vi "Sequence Configurator.vi"() -> ()   [LabVIEW 2024]
doc: "Use this to configure the order of the tests in <project root>/Tests."
uses:
  <vilib>/addons/_JKI Toolkits/State Machine/_JKI_lib_State_Machine.llb/Select State(s)_err__jki_lib_state_machine.vi
  <vilib>/addons/_JKI Toolkits/State Machine/_JKI_lib_State_Machine.llb/Periodic Trigger__ogtk__JKI-SM__jki_lib_state_machine.vi
  <userlib>/_OpenG.lib/file/file.llb/Convert File Extension (String)__ogtk.vi
  <vilib>/Utility/file.llb/Write Delimited Spreadsheet (string).vi
  <userlib>/_OpenG.lib/file/file.llb/openg_file.lvlib
  <userlib>/_OpenG.lib/appcontrol/appcontrol.llb/openg_application_control.lvlib
panel:
  in  "Sequence Name":string
  in  "Close Button":bool
  in  "Save Button":bool
  in  "Test Case Order":i32(listbox)
  out "error out":errorcluster
  in  "error in":errorcluster
  # "SEQUENCE CONFIGURATOR"
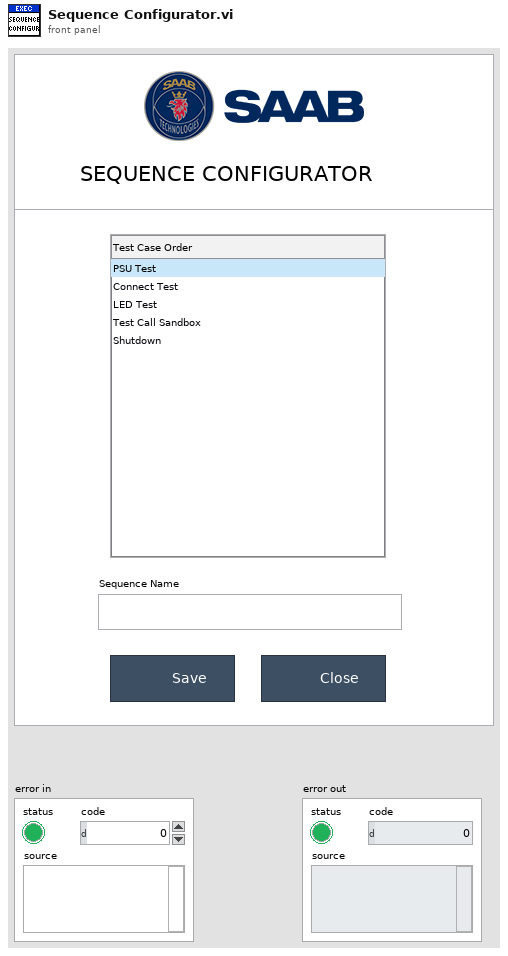
[diagram p1: front panel]
types:
  T1 = enum32{"Invalid", "Standard", "Closed", "Hidden", "Minimized", "Maximized"}
  T2 = enum32{"invalid app kind", "Development System", "Run Time System", "Student Edition", "Embedded LabVIEW", "Evaluation", "Custom"}
  T3 = enum8{"Enabled", "Disabled", "Disabled and Grayed Out"}
  T4 = cluster{"Core":cluster{"Current VI Reference":refnum<vi>, "Close Panel on Exit?":bool}, "Test Case Array":string[], "Sequence Name":string}
  T5 = cluster{"Current VI Reference":refnum<vi>, "Close Panel on Exit?":bool}
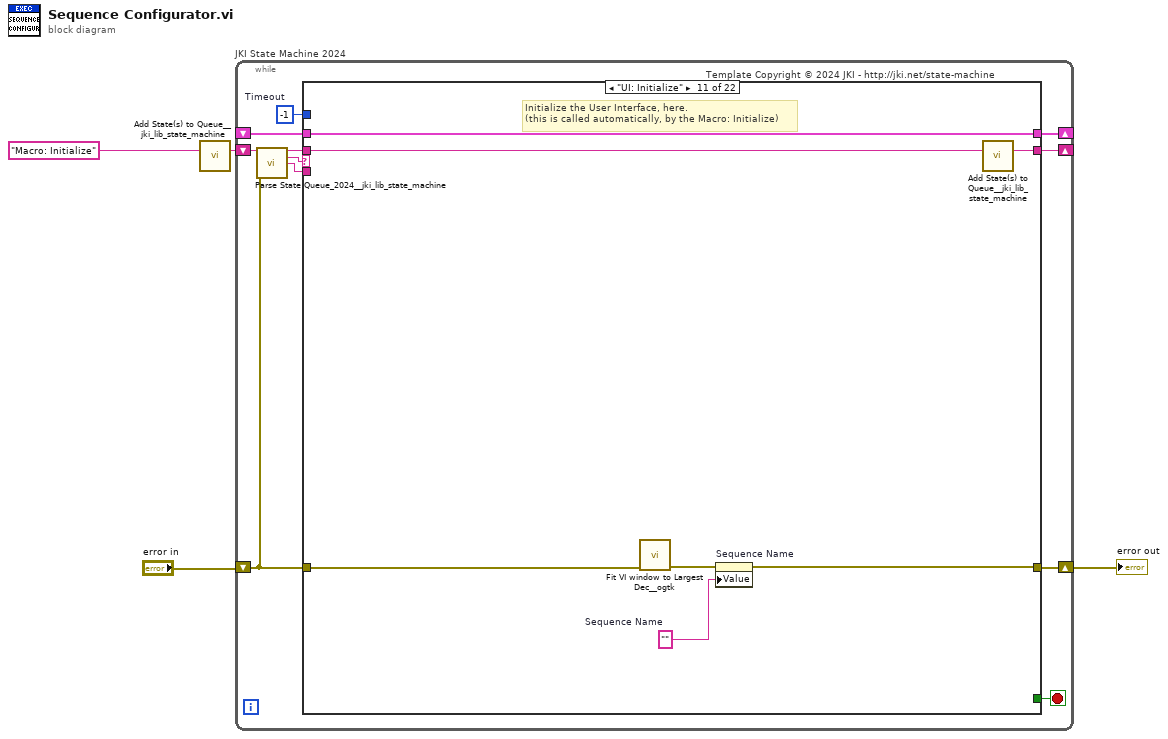
[diagram p0: block diagram]
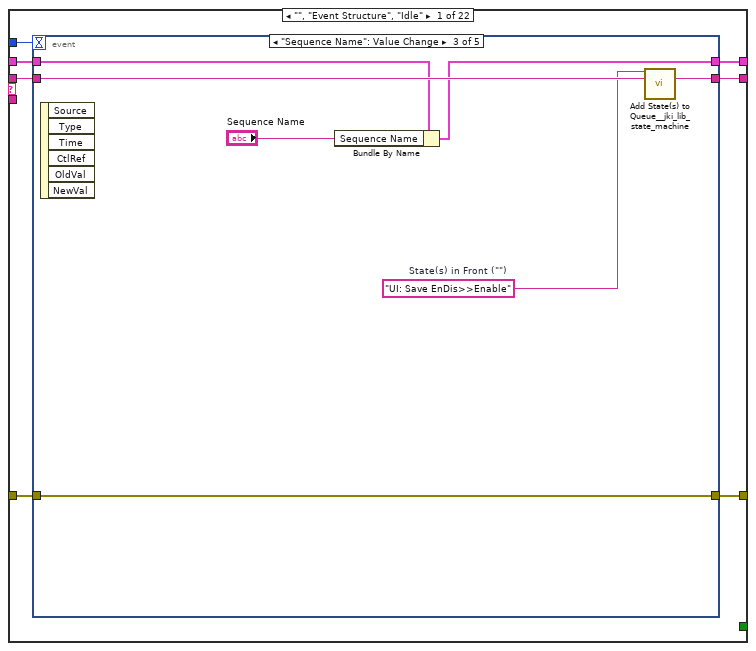
[diagram p2: hidden frame]
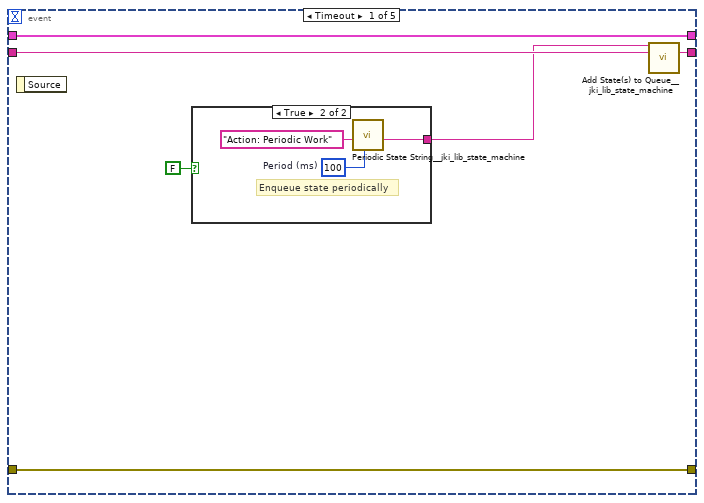
[diagram p3: hidden frame]
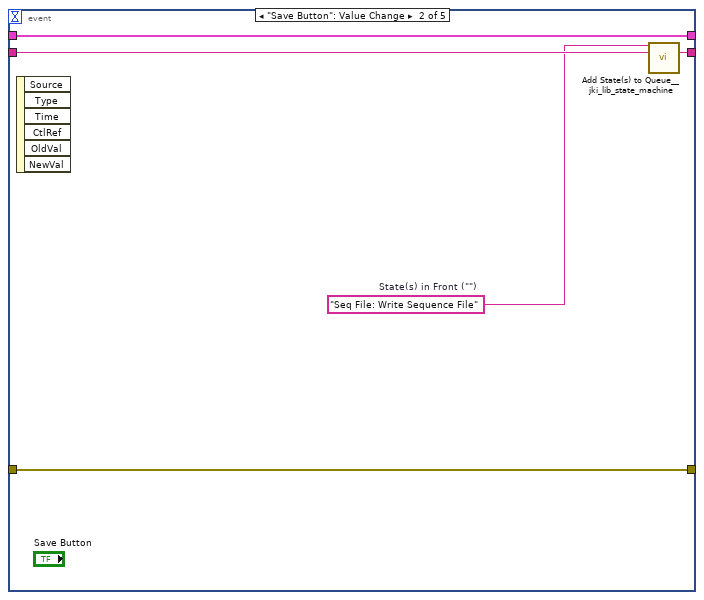
[diagram p5: hidden frame]
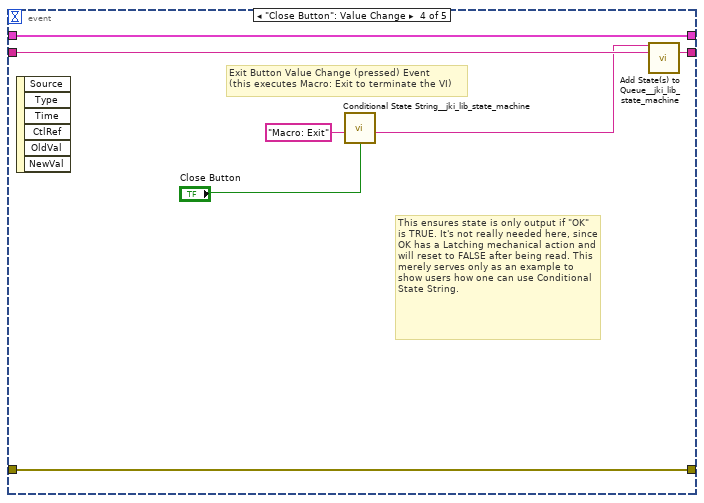
[diagram p6: hidden frame]
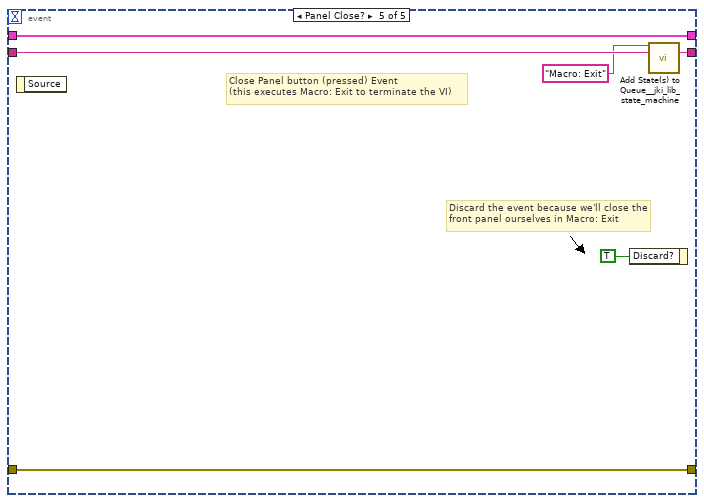
[diagram p7: hidden frame]
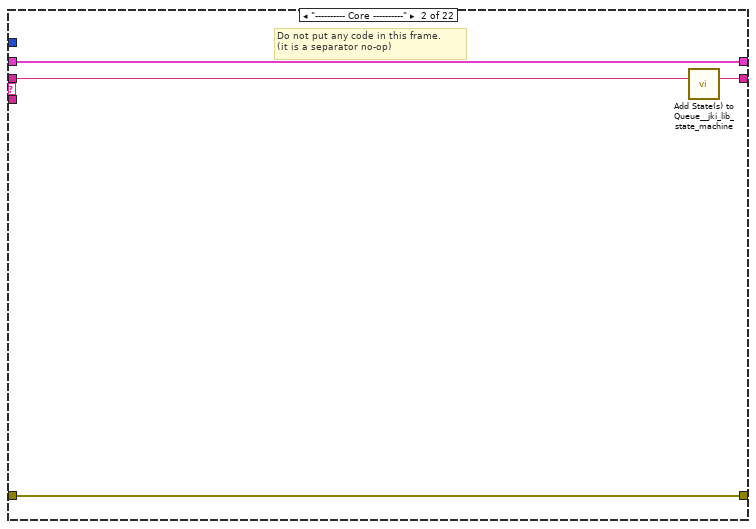
[diagram p8: hidden frame]
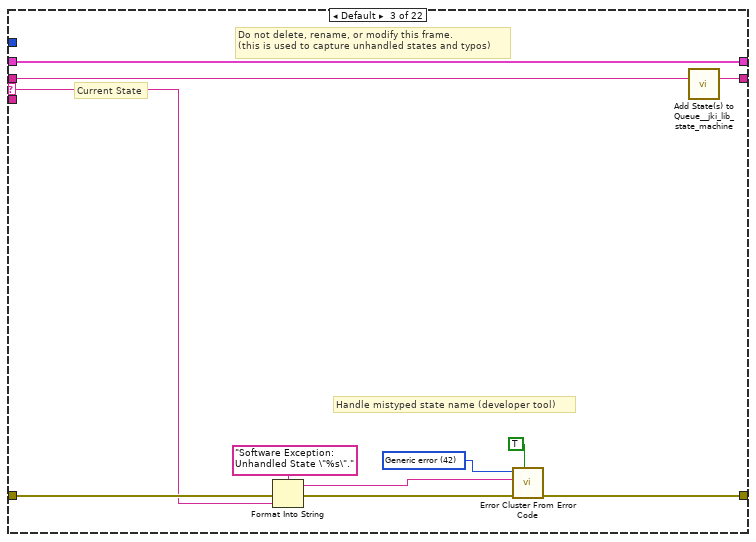
[diagram p9: hidden frame]
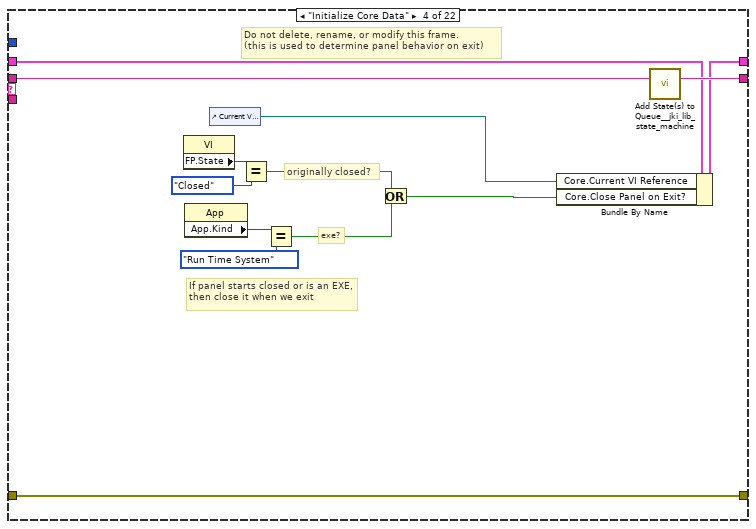
[diagram p10: hidden frame]
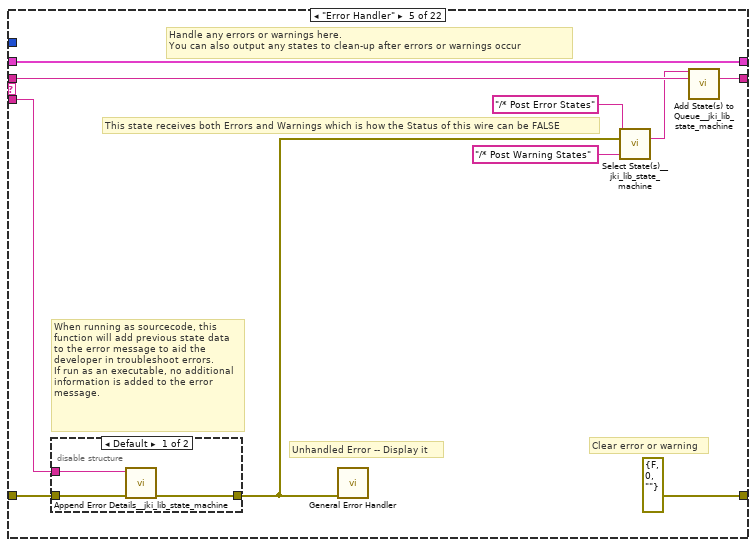
[diagram p11: hidden frame]
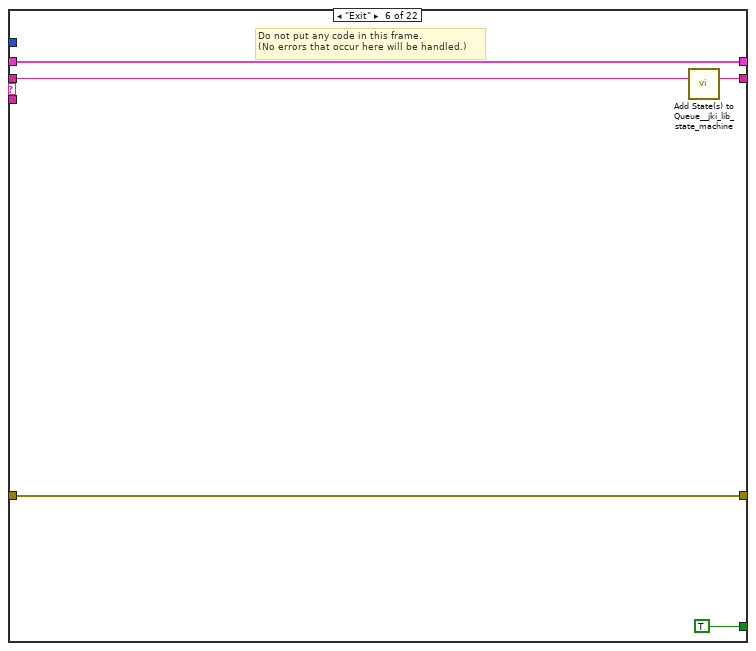
[diagram p13: hidden frame]
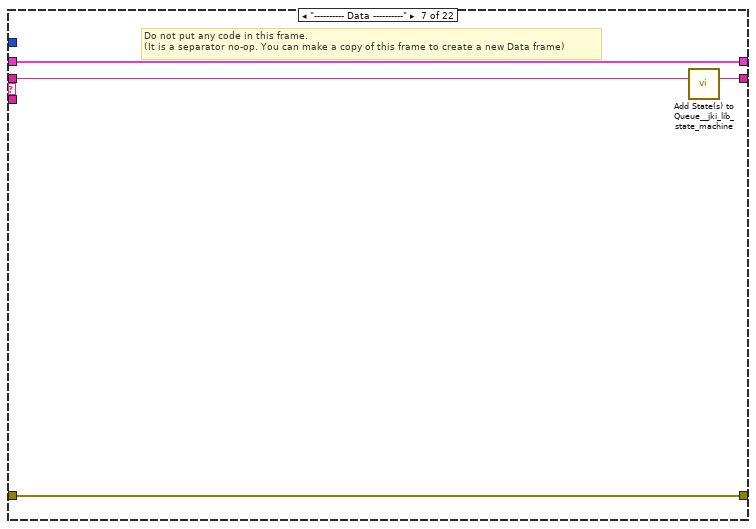
[diagram p14: hidden frame]
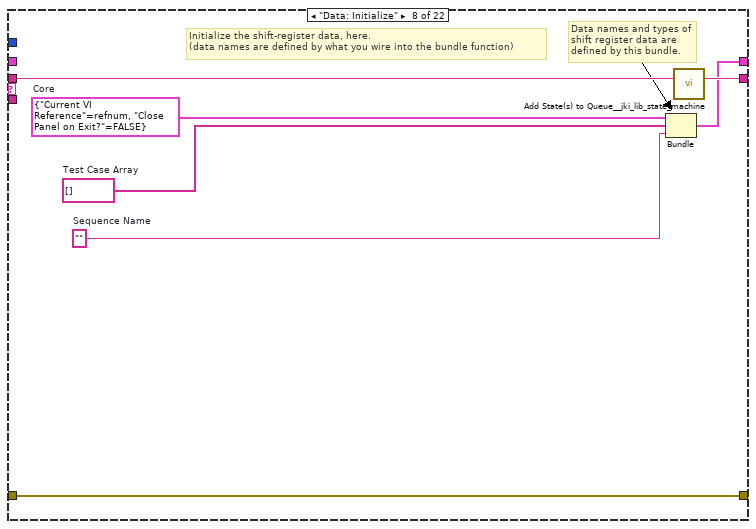
[diagram p15: hidden frame]
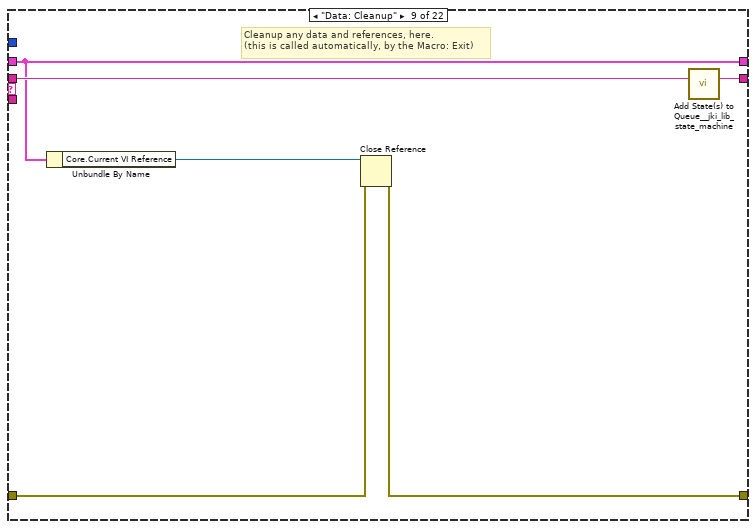
[diagram p16: hidden frame]
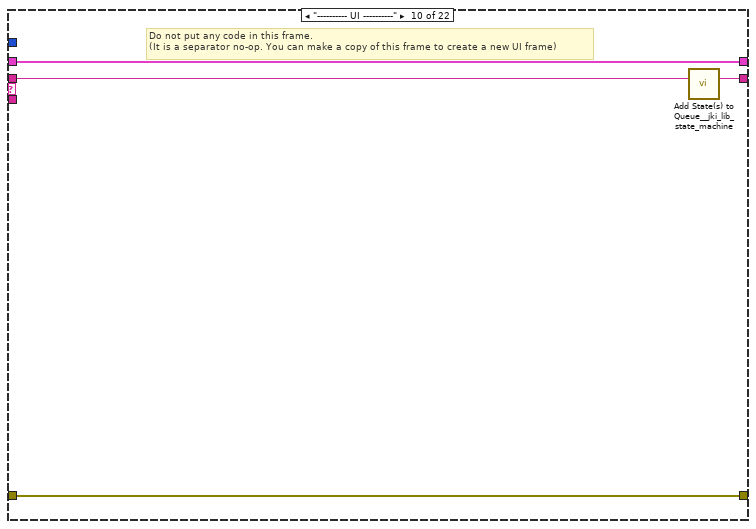
[diagram p17: hidden frame]
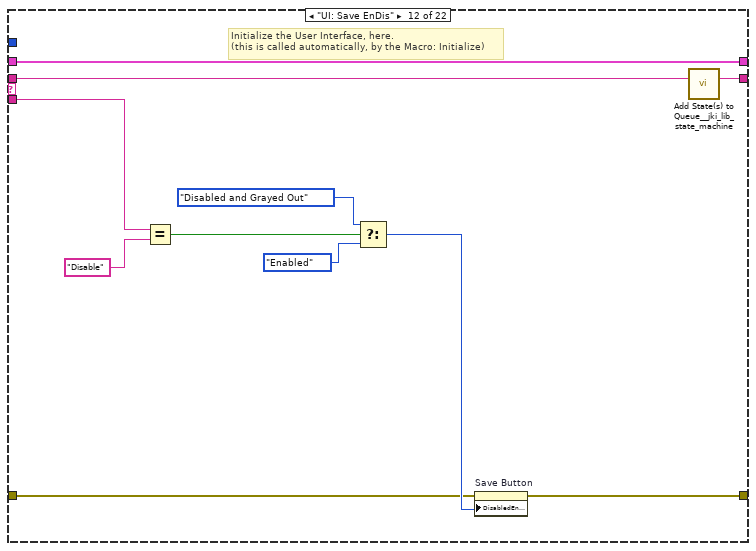
[diagram p18: hidden frame]
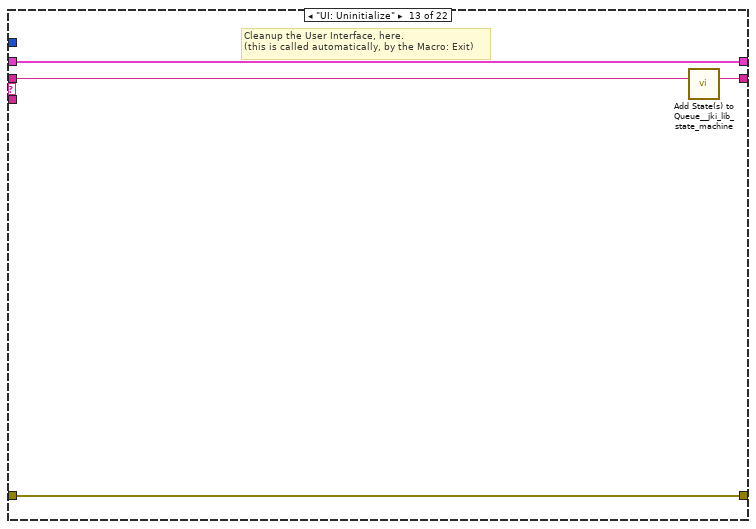
[diagram p19: hidden frame]
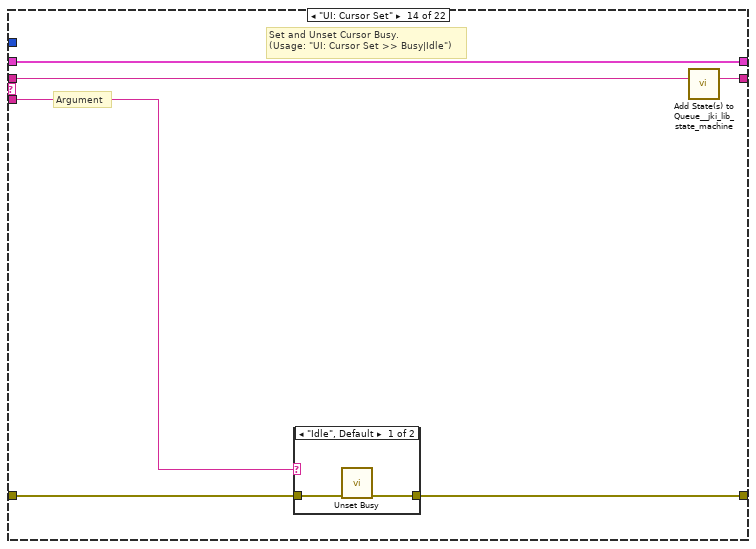
[diagram p20: hidden frame]
diagram:
  n1 = call <vilib>:"Add State(s) to Queue__jki_lib_state_machine.vi"("State(s) in (\"\")"="Macro: Initialize") -> ("States Out"=w4:string)  [unwired: 14 in]
  n2 = while "JKI State Machine 2024" {
    shift-right: [w8] -> _
    shift-left: _ -> [w7]
    shift-right: [w11] -> w1
    shift-left: "error in" -> [w5]
    shift-right: [w10] -> _
    shift-left: w4 -> [w12]
    stop <- w9 stop-if-true
    w6 = -1  # Timeout
    # "Template Copyright © 2024 JKI - http://jki.net/state-machine"
    n3 = call <vilib>:"Parse State Queue_2024__jki_lib_state_machine.vi"("State Queue"=w12, "Error In (no error)"=w5) -> ("Remaining States"=w14:string, "Current State"=w15:string, "Arguments"=w13:string)  [unwired: 11 in]
    n4 = case shown="\"UI: Initialize\"" w15 {
      selector: w15 -> [_ _ w61 _ _ _ _ _ _ _ _ _ _ _ _ _ _ _ _ _ _ _]
      tunnel: w14 -> [w22 w60 w65 w84 w94 w103 w107 w114 w120 w124 w131 w142 w146 w152 w163 w232 w237 w246 w250 w262 w273 w286]
      tunnel: w13 -> [_ _ _ _ w89 _ _ _ _ _ _ w132 _ w147 w157 _ _ _ _ _ _ _]
      tunnel: w7 -> [w20 w57 w63 w77 w91 w101 w104 _ w115 w121 w129 w140 w144 w150 w159 w229 w234 w244 w247 w257 w271 w277]
      tunnel: [w19 w58 w67 w81 errorcluster {"status"=FALSE, "code"=0, "source"=""} ("error out") w100 w105 w111 w116 w122 w127 w133 w143 w148 w160 w230 w235 w241 w248 w260 w266 w282] -> w11
      tunnel: w5 -> [w16 w58 w66 w81 w90 w100 w105 w111 w117 w122 w128 w134 w143 w149 w161 w230 w235 w241 w248 w260 w267 w284]
      tunnel: [w21 w59 w64 w83 w93 w102 w106 w113 w119 w123 w130 w141 w145 w151 w162 w231 w236 w245 w249 w261 w272 w285] -> w10
      tunnel: [_ _ _ _ _ TRUE _ _ _ _ _ _ _ _ _ _ _ _ _ _ _ _] -> w9
      tunnel: [w18 w57 w63 w82 w91 w101 w104 w112 w115 w121 w129 w140 w144 w150 w159 w229 w234 w244 w247 w256 w271 w277] -> w8
      tunnel: w6 -> [w17 _ _ _ _ _ _ _ _ _ _ _ _ _ _ _ _ _ _ _ _ _]
      frame "", "Event Structure", "Idle" {
        n5 = event shown="[2] \"Sequence Name\": Value Change" {
          selector: _ -> [_ _ _ _ _]
          dyn-events: _ -> [_ _ _ _ _]
          timeout: w17 -> [_ _ _ _ _]
          tunnel: w22 -> [w28 w36 w41 w50 w56]
          tunnel: [w27 w35 w42 w49 w55] -> w21
          tunnel: w20 -> [w25 w33 w40 w47 w53]
          tunnel: [w26 w34 w43 w48 w54] -> w19
          tunnel: w16 -> [w26 w34 w43 w48 w54]
          tunnel: [w25 w33 w39 w47 w53] -> w18
          event Timeout {
            n6 = event-data() -> ()  [unwired: 1 in, 1 out]
            n7 = case shown="True" FALSE {
              tunnel: [_ w31] -> w24
              frame False {
              }
              frame True {
                w29 = u32 100  # Period (ms)
                # "Enqueue state periodically"
                n8 = call <vilib>:"Periodic State String__jki_lib_state_machine.vi"("Period (ms)"=w29, "State"="Action: Periodic Work") -> ("State Out"=w31:string)  [unwired: 9 in]
              }
            }
            n9 = call <vilib>:"Add State(s) to Queue__jki_lib_state_machine.vi"("State(s) in Front (\"\")"=w24, "State(s) in (\"\")"=w28) -> ("States Out"=w27:string)  [unwired: 13 in]
          }
          event "Save Button": Value Change {
            w32 = "Seq File: Write Sequence File"  # State(s) in Front ("")
            n10 = event-data() -> ()  [unwired: 1 in, 6 out]
            n11 = call <vilib>:"Add State(s) to Queue__jki_lib_state_machine.vi"("State(s) in Front (\"\")"=w32, "State(s) in (\"\")"=w36) -> ("States Out"=w35:string)  [unwired: 13 in]
          }
          event "Sequence Name": Value Change {
            w37 = "UI: Save EnDis>>Enable"  # State(s) in Front ("")
            n12 = event-data() -> ()  [unwired: 1 in, 6 out]
            n13 = Bundle By Name(cluster=w40, "Sequence Name"="Sequence Name") -> (w39:T4)
            n14 = call <vilib>:"Add State(s) to Queue__jki_lib_state_machine.vi"("State(s) in Front (\"\")"=w37, "State(s) in (\"\")"=w41) -> ("States Out"=w42:string)  [unwired: 13 in]
          }
          event "Close Button": Value Change {
            # "This ensures state is only output if \"OK\" is TRUE. It's not really needed here, since OK has a Latching mechanical action and will reset to FALSE after being read. This merely serves only as an example to show users how one can use Conditional State String."
            # "Exit Button Value Change (pressed) Event\n(this executes Macro: Exit to terminate the VI)"
            n15 = event-data() -> ()  [unwired: 1 in, 6 out]
            n16 = call <vilib>:"Conditional State String__jki_lib_state_machine.vi"("Do State(s)?"="Close Button", "State"="Macro: Exit") -> ("State Out"=w45:string)  [unwired: 7 in]
            n17 = call <vilib>:"Add State(s) to Queue__jki_lib_state_machine.vi"("State(s) in Front (\"\")"=w45, "State(s) in (\"\")"=w50) -> ("States Out"=w49:string)  [unwired: 13 in]
          }
          event Panel Close? {
            # "Discard the event because we'll close the front panel ourselves in Macro: Exit"
            # "Close Panel button (pressed) Event\n(this executes Macro: Exit to terminate the VI)"
            n18 = event-data() -> ()  [unwired: 1 in, 1 out]
            n19 = event-data("Discard?"=TRUE) -> ()  [unwired: 1 in, 1 out]
            n20 = call <vilib>:"Add State(s) to Queue__jki_lib_state_machine.vi"("State(s) in Front (\"\")"="Macro: Exit", "State(s) in (\"\")"=w56) -> ("States Out"=w55:string)  [unwired: 13 in]
          }
        }
      }
      frame "---------- Core ----------" {
        # "Do not put any code in this frame.\n(it is a separator no-op)"
        n21 = call <vilib>:"Add State(s) to Queue__jki_lib_state_machine.vi"("State(s) in (\"\")"=w60) -> ("States Out"=w59:string)  [unwired: 14 in]
      }
      frame Default {
        w70 = 42 items=["No error", "Argument error", "Memory is full", "Out of zone", "End of file", "File already open", "Generic file I/O error", "File not found", "File permission error", "Disk is full", "Duplicate path", "Too many files open", "System feature not enabled", "Resource file not found", "Cannot add resource", "Resource not found", "Image not found", "Image memory error", "Pen does not exist", "Config type invalid", "Config token not found", "Config parse error", "Config memory error", "Bad external code format", "Bad external code offset", "External code not present", "Null window", "Destroy window error", "Null menu", "Print aborted", "Bad print record", "Print driver error", "Windows error during printing", "Memory error during printing", "Print dialog error", "Generic print error", "Invalid device refnum", "Device not found", "Device parameter error", "Device unit error", "Cannot open device", "Device call aborted", "Generic error", "Cancelled by user", "Object ID too low", "Object ID too high", "Object not in heap", "Unknown heap", "Unknown object (invalid DefProc)", "Unknown object (DefProc not in table)", "Message out of range", "Invalid (null) method", "Unknown message", "Manager call not supported", "Bad address", "Network operation in progress", "Network operation timed out", "Connection is busy", "Network attribute not supported", "Network error", "Address in use", "System out of memory", "Connection aborted", "Connection refused", "Not connected", "Already connected", "Connection closed", "Initialization error (interapplication manager)", "Bad occurrence", "Wait on unbound occurrence handler", "Occurrence queue overflow", "Datalog type conflict", "Unused", "Unrecognized type (interapplication manager)", "Memory corrupt", "Failed to make temporary DLL", "Old CIN version", "Drag socket not found", "Failed to load drop-object", "Failed to register OLE object", "Failed to release OLE object", "Format specifier type mismatch", "Unknown format specifier", "Too few format specifiers", "Too many format specifiers", "Scan failed", "Newer CIN version", "Error converting to variant", "Runtime menu error", "Password tampered", "Variant attribute not found", "Incompatible variant data type", "Event data is not available", "Event Store is not present", "Occurrence is not found", "Event Queue is not created", "Event info is not available", "Refnum passed is NULL", "Error retrieving Class GUID", "Error retrieving CoClass GUID", "Error retrieving TypeLib GUID.", "Bad built application magic bytes.", "Specific driver is different from the specific driver associated with the Logical Name.", "There is no session opened to the class driver.", "Max Error", "MAX - Error with config objects", "MAX - Error loading configuration", "MAX - Group not supported"]
        # "Current State"
        # "Do not delete, rename, or modify this frame.\n(this is used to capture unhandled states and typos)"
        # "Handle mistyped state name (developer tool)"
        n22 = Format Into String(format string="Software Exception: Unhandled State \"%s\"." ("message"), error in=w66, w61) -> (resulting string=w69:string, error out=w68:errorcluster)  [unwired: 1 in]
        n23 = call <vilib>:"Error Cluster From Error Code.vi"("show call chain? (False)"=TRUE, "error in (no error)"=w68, "error message (\"\")"=w69, "error code (0)"=w70) -> ("error out"=w67:errorcluster)  [unwired: 5 in]
        n24 = call <vilib>:"Add State(s) to Queue__jki_lib_state_machine.vi"("State(s) in (\"\")"=w65) -> ("States Out"=w64:string)  [unwired: 14 in]
      }
      frame "Initialize Core Data" {
        # "Do not delete, rename, or modify this frame.\n(this is used to determine panel behavior on exit)"
        # "originally closed?"
        # "exe?"
        # "If panel starts closed or is an EXE, then close it when we exit"
        n25 = property class="VI"() -> ("FP.State"=w74:T1)  [unwired: 2 in, 2 out]
        n26 = property class="App"() -> ("App.Kind"=w80:T2)  [unwired: 2 in, 2 out]
        n27 = control-ref of="Current VI Reference"() -> (w75:refnum<vi>)
        n28 = Equal?(x=w74, y=T1."Closed" ("Front Panel Window:State")) -> (x = y?=w72:bool)
        n29 = Equal?(x=w80, y=T2."Run Time System" ("Application:Kind")) -> (x = y?=w78:bool)
        n30 = Or(x=w72, y=w78) -> (x .or. y?=w76:bool)
        n31 = Bundle By Name(cluster=w77, "Core.Current VI Reference"=w75, "Core.Close Panel on Exit?"=w76) -> (w82:T4)
        n32 = call <vilib>:"Add State(s) to Queue__jki_lib_state_machine.vi"("State(s) in (\"\")"=w84) -> ("States Out"=w83:string)  [unwired: 14 in]
      }
      frame "Error Handler" {
        # "When running as sourcecode, this function will add previous state data to the error message to aid the developer in troubleshoot errors.\nIf run as an executable, no additional information is added to the error message."
        # "This state receives both Errors and Warnings which is how the Status of this wire can be FALSE"
        # "Unhandled Error -- Display it"
        # "Handle any errors or warnings here.\nYou can also output any states to clean-up after errors or warnings occur"
        # "Clear error or warning"
        n33 = disable-structure shown="Default" {
          disable-tunnel: w90 -> [w97 w98]
          disable-tunnel: w89 -> [w96 _]
          disable-tunnel: [w95 w98] -> w88
          frame condition #0 (active) {
            n34 = call <vilib>:"Append Error Details__jki_lib_state_machine.vi"("error in (no error)"=w97, "Previous State and Argument(s)"=w96) -> ("error out"=w95:errorcluster)  [unwired: 9 in]
          }
          frame condition #1 {
          }
        }
        n35 = call <vilib>:"General Error Handler.vi"("error in (no error)"=w88) -> ()  [unwired: 10 in, 5 out]
        n36 = call-poly <vilib>:"Select State(s)__jki_lib_state_machine.vi"("State(s) if True (\"\")"="/* Post Error States", "Select"=w88, "State(s) if False (\"\")"="/* Post Warning States") -> ("States Out"=w86:string)  [unwired: 12 in]
        n37 = call <vilib>:"Add State(s) to Queue__jki_lib_state_machine.vi"("State(s) in Front (\"\")"=w86, "State(s) in (\"\")"=w94) -> ("States Out"=w93:string)  [unwired: 13 in]
      }
      frame "Exit" {
        # "Do not put any code in this frame.\n(No errors that occur here will be handled.)"
        n38 = call <vilib>:"Add State(s) to Queue__jki_lib_state_machine.vi"("State(s) in (\"\")"=w103) -> ("States Out"=w102:string)  [unwired: 14 in]
      }
      frame "---------- Data ----------" {
        # "Do not put any code in this frame.\n(It is a separator no-op. You can make a copy of this frame to create a new Data frame)"
        n39 = call <vilib>:"Add State(s) to Queue__jki_lib_state_machine.vi"("State(s) in (\"\")"=w107) -> ("States Out"=w106:string)  [unwired: 14 in]
      }
      frame "Data: Initialize" {
        w108 = ""  # Sequence Name
        w109 = string[] []  # Test Case Array
        w110 = T5 {"Current VI Reference"=refnum, "Close Panel on Exit?"=FALSE}  # Core
        # "Data names and types of shift register data are defined by this bundle."
        # "Initialize the shift-register data, here.\n(data names are defined by what you wire into the bundle function)"
        n40 = Bundle("Core"=w110, "Test Case Array"=w109, "Sequence Name"=w108) -> (w112:T4)  [unwired: 1 in]
        n41 = call <vilib>:"Add State(s) to Queue__jki_lib_state_machine.vi"("State(s) in (\"\")"=w114) -> ("States Out"=w113:string)  [unwired: 14 in]
      }
      frame "Data: Cleanup" {
        # "Cleanup any data and references, here.\n(this is called automatically, by the Macro: Exit)"
        n42 = Unbundle By Name(w115) -> ("Core.Current VI Reference"=w118:refnum<vi>)
        n43 = Close Reference(reference=w118, error in (no error)=w117) -> (error out=w116:errorcluster)
        n44 = call <vilib>:"Add State(s) to Queue__jki_lib_state_machine.vi"("State(s) in (\"\")"=w120) -> ("States Out"=w119:string)  [unwired: 14 in]
      }
      frame "---------- UI ----------" {
        # "Do not put any code in this frame.\n(It is a separator no-op. You can make a copy of this frame to create a new UI frame)"
        n45 = call <vilib>:"Add State(s) to Queue__jki_lib_state_machine.vi"("State(s) in (\"\")"=w124) -> ("States Out"=w123:string)  [unwired: 14 in]
      }
      frame "UI: Initialize" {
        w125 = ""  # Sequence Name
        # "Initialize the User Interface, here.\n(this is called automatically, by the Macro: Initialize)"
        n46 = call <userlib>:"Fit VI window to Largest Dec__ogtk.vi"("error in (no error)"=w128) -> ("error out"=w126:errorcluster)  [unwired: 5 in, 1 out]
        n47 = property on="Sequence Name" class="Str"(error in=w126, "Value"=w125) -> (error out=w127:errorcluster)  [unwired: 1 in, 1 out]
        n48 = call <vilib>:"Add State(s) to Queue__jki_lib_state_machine.vi"("State(s) in (\"\")"=w131) -> ("States Out"=w130:string)  [unwired: 14 in]
      }
      frame "UI: Save EnDis" {
        # "Initialize the User Interface, here.\n(this is called automatically, by the Macro: Initialize)"
        n49 = Equal?(x=w132, y="Disable") -> (x = y?=w135:bool)
        n50 = Select(t=T3."Disabled and Grayed Out" ("Disabled"), s=w135, f=T3."Enabled" ("Disabled")) -> (s? t:f=w136:T3)
        n51 = property on="Save Button" class="Bool"(error in=w134, "DisabledEnum"=w136) -> (error out=w133:errorcluster)  [unwired: 1 in, 1 out]
        n52 = call <vilib>:"Add State(s) to Queue__jki_lib_state_machine.vi"("State(s) in (\"\")"=w142) -> ("States Out"=w141:string)  [unwired: 14 in]
      }
      frame "UI: Uninitialize" {
        # "Cleanup the User Interface, here.\n(this is called automatically, by the Macro: Exit)"
        n53 = call <vilib>:"Add State(s) to Queue__jki_lib_state_machine.vi"("State(s) in (\"\")"=w146) -> ("States Out"=w145:string)  [unwired: 14 in]
      }
      frame "UI: Cursor Set" {
        # "Argument"
        # "Set and Unset Cursor Busy.\n(Usage: \"UI: Cursor Set >> Busy|Idle\")"
        n54 = case shown="\"Idle\", Default" w147 {
          tunnel: w149 -> [w154 w156]
          tunnel: [w153 w155] -> w148
          frame "Idle", Default {
            n55 = call <vilib>:"Unset Busy.vi"("error in (no error)"=w154) -> ("error out"=w153:errorcluster)  [unwired: 10 in]
          }
          frame "Busy" {
            n56 = call <vilib>:"Set Busy.vi"("error in (no error)"=w156) -> ("error out"=w155:errorcluster)  [unwired: 9 in, 1 out]
          }
        }
        n57 = call <vilib>:"Add State(s) to Queue__jki_lib_state_machine.vi"("State(s) in (\"\")"=w152) -> ("States Out"=w151:string)  [unwired: 14 in]
      }
      frame "UI: Front Panel State" {
        # "Argument"
        # "Set Front Panel Open or Closed\n(Usage: \"UI: Front Panel State >> Open|Close\")"
        n58 = Unbundle By Name(w159) -> ("Core.Current VI Reference"=w158:refnum<vi>)
        n59 = case shown="\"Minimize\", \"Minimized\"" w157 {
          tunnel: w161 -> [w169 w184 w195 w208 w221]
          tunnel: [w171 w185 w197 w210 w223] -> w160
          tunnel: w158 -> [w170 w182 w196 w209 w222]
          frame "Open", "Standard", Default {
            w164 = T1."Standard" ("State")
            n60 = property class="VI"(reference=w170, error in=w169) -> (reference out=w167:refnum<vi>, error out=w168:errorcluster, "FP.State"=w166:T1)
            n61 = Not Equal?(x=w166, y=w164) -> (x != y?=w165:bool)
            n62 = case shown="True" w165 {
              tunnel: [w175 w177] -> w171
              tunnel: w168 -> [w174 w177]
              tunnel: w167 -> [w173 _]
              tunnel: w164 -> [w172 _]
              frame True {
                n63 = invoke class="VI" method="FP.Open"(reference=w173, error in=w174, "Activate"=TRUE, "State"=w172) -> (error out=w175:errorcluster)  [unwired: 1 in, 4 out]
              }
              frame False {
              }
            }
          }
          frame "Close", "Closed" {
            n64 = property class="VI"(reference=w182, error in=w184) -> (reference out=w181:refnum<vi>, error out=w183:errorcluster, "FP.State"=w179:T1)
            n65 = Not Equal?(x=w179, y=T1."Closed" ("Front Panel Window:State")) -> (x != y?=w178:bool)
            n66 = case shown="True" w178 {
              tunnel: [w186 w189] -> w185
              tunnel: w183 -> [w186 w188]
              tunnel: w181 -> [_ w187]
              frame False {
              }
              frame True {
                n67 = invoke class="VI" method="FP.Close"(reference=w187, error in=w188) -> (error out=w189:errorcluster)  [unwired: 1 in, 2 out]
              }
            }
          }
          frame "Hidden", "Hide" {
            w190 = T1."Hidden" ("State")
            n68 = property class="VI"(reference=w196, error in=w195) -> (reference out=w193:refnum<vi>, error out=w194:errorcluster, "FP.State"=w192:T1)
            n69 = Not Equal?(x=w192, y=w190) -> (x != y?=w191:bool)
            n70 = case shown="True" w191 {
              tunnel: [w201 w202] -> w197
              tunnel: w194 -> [w200 w202]
              tunnel: w193 -> [w199 _]
              tunnel: w190 -> [w198 _]
              frame True {
                n71 = invoke class="VI" method="FP.Open"(reference=w199, error in=w200, "State"=w198) -> (error out=w201:errorcluster)  [unwired: 2 in, 4 out]
              }
              frame False {
              }
            }
          }
          frame "Minimize", "Minimized" {
            w203 = T1."Minimized" ("State")
            n72 = property class="VI"(reference=w209, error in=w208) -> (reference out=w206:refnum<vi>, error out=w207:errorcluster, "FP.State"=w205:T1)
            n73 = Not Equal?(x=w205, y=w203) -> (x != y?=w204:bool)
            n74 = case shown="True" w204 {
              tunnel: [w214 w215] -> w210
              tunnel: w207 -> [w213 w215]
              tunnel: w206 -> [w212 _]
              tunnel: w203 -> [w211 _]
              frame True {
                n75 = invoke class="VI" method="FP.Open"(reference=w212, error in=w213, "State"=w211) -> (error out=w214:errorcluster)  [unwired: 2 in, 4 out]
              }
              frame False {
              }
            }
          }
          frame "Maximize", "Maximized" {
            w216 = T1."Maximized" ("State")
            n76 = property class="VI"(reference=w222, error in=w221) -> (reference out=w219:refnum<vi>, error out=w220:errorcluster, "FP.State"=w218:T1)
            n77 = Not Equal?(x=w218, y=w216) -> (x != y?=w217:bool)
            n78 = case shown="True" w217 {
              tunnel: [w227 w228] -> w223
              tunnel: w220 -> [w226 w228]
              tunnel: w219 -> [w225 _]
              tunnel: w216 -> [w224 _]
              frame True {
                n79 = invoke class="VI" method="FP.Open"(reference=w225, error in=w226, "State"=w224) -> (error out=w227:errorcluster)  [unwired: 2 in, 4 out]
              }
              frame False {
              }
            }
          }
        }
        n80 = call <vilib>:"Add State(s) to Queue__jki_lib_state_machine.vi"("State(s) in (\"\")"=w163) -> ("States Out"=w162:string)  [unwired: 14 in]
      }
      frame "---------- Macro ----------" {
        # "Do not put any code in this frame.\n(It is a separator no-op. You can make a copy of this frame to create a new Macro frame)"
        n81 = call <vilib>:"Add State(s) to Queue__jki_lib_state_machine.vi"("State(s) in (\"\")"=w232) -> ("States Out"=w231:string)  [unwired: 14 in]
      }
      frame "Macro: Initialize" {
        w233 = "Data: Initialize\nInitialize Core Data\nUI: Initialize\nUI: Save EnDis>>Disable\nUI: Front Panel State >> Open\nSeq File: Test Case Folder\nSeq File: Populate Listbox"  # Data: Initialize Initialize Core Data UI: Initialize UI: Save EnDis>>Disable UI: Front Panel State >> Open Seq File: Test Case Folder Seq File: Populate Listbox
        # "Initialization Macro\n(This is called once, when the VI starts)"
        n82 = call <vilib>:"Add State(s) to Queue__jki_lib_state_machine.vi"("State(s) in Front (\"\")"=w233, "State(s) in (\"\")"=w237) -> ("States Out"=w236:string)  [unwired: 13 in]
      }
      frame "Macro: Exit" {
        # "Exit Macro\n(This is called once, when the VI exits)"
        n83 = Unbundle By Name(w244) -> ("Core.Close Panel on Exit?"=w239:bool)
        n84 = call <vilib>:"Conditional State String__jki_lib_state_machine.vi"("Do State(s)?"=w239, "State"="UI: Front Panel State >> Close") -> ("State Out"=w238:string)  [unwired: 7 in]
        n85 = call <vilib>:"Add State(s) to Queue__jki_lib_state_machine.vi"("State(s) in (\"\")"=w238, "State(s) at Back (\"\")"="UI: Uninitialize\nData: Cleanup\nExit") -> ("States Out"=w242:string)  [unwired: 13 in]
        n86 = call <vilib>:"Add State(s) to Queue__jki_lib_state_machine.vi"("State(s) in Front (\"\")"=w242, "State(s) in (\"\")"=w246) -> ("States Out"=w245:string)  [unwired: 13 in]
      }
      frame "---------- Seq File ----------" {
        # "Template Separator\n(You can make a copy of, or modify, this frame)"
        n87 = call <vilib>:"Add State(s) to Queue__jki_lib_state_machine.vi"("State(s) in (\"\")"=w250) -> ("States Out"=w249:string)  [unwired: 14 in]
      }
      frame "Seq File: Test Case Folder" {
        w259 = "*.vi"  # pattern
        n88 = call <userlib>:"Current VIs Parent Directory__ogtk.vi"() -> ("Parent Directory (+ Relative)"=w252:path)  [unwired: 5 in]
        n89 = Strip Path(path=w252) -> (stripped path=w251:path)  [unwired: 1 out]
        n90 = Build Path(base path=w251, name or relative path="Tests") -> (appended path=w253:path)
        n91 = List Folder(path=w253, pattern=w259) -> (filenames=w258:string[])  [unwired: 2 in, 3 out]
        n92 = for {
          tunnel: w258 -> [w264] mode=indexing
          tunnel: [w263] -> w255 mode=indexing
          n93 = call-poly <userlib>:"Convert File Extension__ogtk.vi"("file name"=w264) -> ("new filename"=w263:string)  [unwired: 1 in, 1 out]
        }
        n94 = Bundle By Name(cluster=w257, "Test Case Array"=w255) -> (w256:T4)
        n95 = call <vilib>:"Add State(s) to Queue__jki_lib_state_machine.vi"("State(s) in (\"\")"=w262) -> ("States Out"=w261:string)  [unwired: 14 in]
      }
      frame "Seq File: Populate Listbox" {
        w268 = TRUE  # Drag/Drop:Allow Dragging
        w270 = "Test Case Order"  # Column Header String
        n96 = Unbundle By Name(w271) -> ("Test Case Array"=w265:string[])
        n97 = property on="Test Case Order" class="LstBox (strict)"(error in=w267, "Item Names"=w265, "ColHdr"=w270) -> (error out=w269:errorcluster)  [unwired: 1 in, 1 out]
        n98 = property on="Test Case Order" class="LstBox (strict)"(error in=w269, "Allow Item Drag"=w268, "Allow Drop"=w268) -> (error out=w266:errorcluster)  [unwired: 1 in, 1 out]
        n99 = call <vilib>:"Add State(s) to Queue__jki_lib_state_machine.vi"("State(s) in (\"\")"=w273) -> ("States Out"=w272:string)  [unwired: 14 in]
      }
      frame "Seq File: Write Sequence File" {
        w275 = ".csv"  # string
        w280 = ","  # delimiter (\t)
        # "Your code here.\n(You can make a copy of, or modify, this frame)"
        n100 = Unbundle By Name(w277) -> ("Sequence Name"=w276:string)
        n101 = property on="Test Case Order" class="LstBox (strict)"(error in=w284) -> (error out=w283:errorcluster, "Item Names"=w281:string[])  [unwired: 1 in, 1 out]
        n102 = Concatenate Strings(w276, w275) -> (w274:string)
        n103 = call <userlib>:"Current VIs Parent Directory__ogtk.vi"() -> ("Parent Directory (+ Relative)"=w279:path)  [unwired: 5 in]
        n104 = Build Path(base path=w279, name or relative path=w274) -> (appended path=w278:path)
        n105 = call-poly <vilib>:"Write Delimited Spreadsheet.vi"("file path (dialog if empty)"=w278, "1D data"=w281, "error in (no error)"=w283, "delimiter (\\t)"=w280) -> ("error out"=w282:errorcluster)  [unwired: 10 in, 1 out]
        n106 = call <vilib>:"Add State(s) to Queue__jki_lib_state_machine.vi"("State(s) in (\"\")"=w286) -> ("States Out"=w285:string)  [unwired: 14 in]
      }
    }
  }
  "error out" <- w1
